vi "Get RPC Type.vi"(1 "RPC Method Parameters":T2) -> (0 "RPC Type":T1)   [LabVIEW 2019, in "gRPC Template Creation Utility.lvlib"]
uses:
  gRPC Template Creation Utility.lvlib
  TypeDefs/RPC Method Parameters.ctl
  TypeDefs/RPC Method Types.ctl
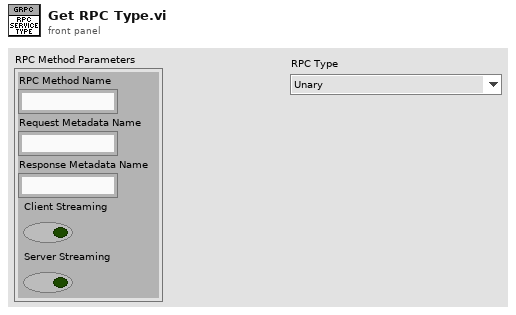
[diagram p1: front panel]
types:
  T1 = typedef "gRPC Template Creation Utility.lvlib/RPC Method Types.ctl" = enum16{"Unary", "Server Stream", "Client Stream", "Bidirectional Stream"}
  T2 = typedef "gRPC Template Creation Utility.lvlib/RPC Method Parameters.ctl" = cluster{"RPC Method Name":string, "Request Metadata Name":string, "Response Metadata Name":string, "Client Streaming":bool, "Server Streaming":bool}
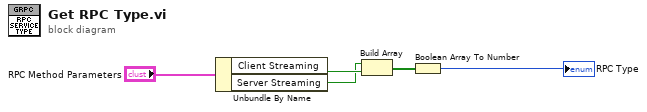
[diagram p0: block diagram]
diagram:
  n1 = Unbundle By Name("RPC Method Parameters") -> ("Client Streaming"=w4:bool, "Server Streaming"=w3:bool)
  n2 = Build Array(w3, w4) -> (w2:bool[])
  n3 = Boolean Array To Number(Boolean array=w2) -> (number=→"RPC Type":u32)
